vi "disabled from Main.vi"   [LabVIEW 2020]
uses:
  controls/step_type.ctl
  controls/PROTO_stepV2.ctl
  controls/visa resource names.ctl
types:
  T1 = typedef "visa resource names.ctl" = enum16{"12V power supply 1", "12V power supply 2", "Chroma 19053 HIPOT", "Chroma 62150 100V/3kw DCDC Load", "Chroma 62150 500V 50kw Power Supply", "Chroma 17040 regen battery", "Chroma 63205 compressor electric load", "Chroma 63208 heater electric load", ""}
  T2 = typedef "PROTO_stepV2.ctl" = cluster{"VISA resource name":string, "data num":dbl, "step_description (prompt)":string, "step_json":string, "save results":bool, "step_type":T3, "Step_name":string, "data bool":bool}
  T3 = typedef "step_type.ctl" = enum16{"default", "prompt", "sequence#", "12V_1_power supply on_off", "12V_2_power supply on_off", "set_hipot_V", "set_hipot_I_limit", "set_hipot_ramping (sec)", "set hipot_hold_time", "read_hipot_V", "read_hipot_I", "set_daq", "read_daq", "flash uds", "wait (sec)", "record_pass_fail", "ac_charge_test", "dc_400V_charging", "HAPS Heater Output", "HAPS Compressor Output", "stop_test", "error_exit"}
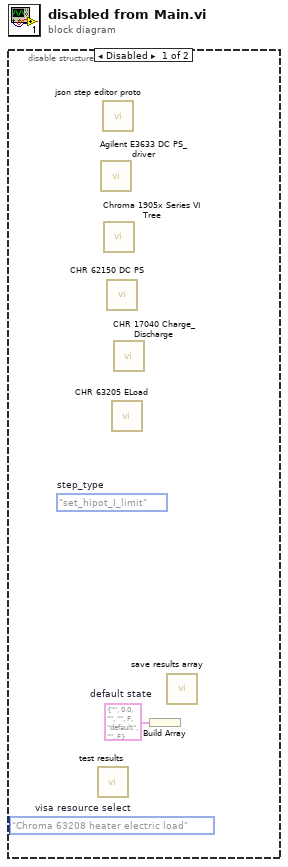
[diagram p0: block diagram]
diagram:
  n1 = disable-structure shown="Disabled" {
    frame Disabled {
      (unwired) visa_resource_names."Chroma 63208 heater electric load"  # visa resource select
      w1 = T2 {"VISA resource name"="", "data num"=0.0, "step_description (prompt)"="", "step_json"="", "save results"=FALSE, "step_type"=enum."default", "Step_name"="", "data bool"=FALSE}  # default state
      (unwired) step_type."set_hipot_I_limit"  # step_type
      n2 = call "test results.vi"() -> ()  [unwired: 11 in, 1 out]
      n3 = call "Agilent E3633 DC PS_driver.vi"() -> ()  [unwired: 8 in, 4 out]
      n4 = call "json step editor proto.vi"() -> ()  [unwired: 12 in]
      n5 = call <instrlib>:"Chroma 1905x Series VI Tree.vi"() -> ()  [unwired: 1 in]
      n6 = call "CHR 62150 DC PS.vi"() -> ()  [unwired: 12 in]
      n7 = call "CHR 63205 ELoad.vi"() -> ()  [unwired: 12 in]
      n8 = call "CHR 17040 Charge_Discharge.vi"() -> ()  [unwired: 12 in]
      n9 = Build Array(w1) -> ()  [unwired: 1 out]
      n10 = call "save results array.vi"() -> ()  [unwired: 11 in, 1 out]
    }
    frame Enabled {
    }
  }
